vi "_complementStringArrays.vi"(9 "B":string[](array[string]), 10 "A":string[](array[string])) -> (2 "Result":string[](array[string]))   [LabVIEW 2013, in "tWorkerController.lvlib" / "tWorkerController.lvclass"]
doc: "Returns elements from A that don't exist in B."
uses:
  tWorkerController.lvclass
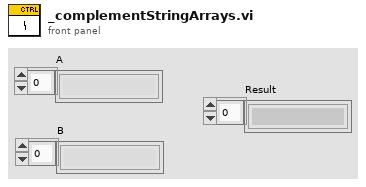
[diagram p1: front panel]
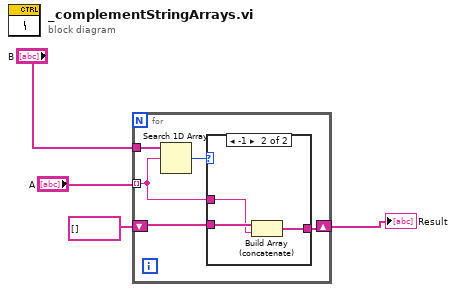
[diagram p0: block diagram]
diagram:
  n1 = for {
    tunnel: "A" -> [w7] mode=indexing
    shift-right: [w5] -> w1
    shift-left: string[] [] -> [w6]
    tunnel: "B" -> [w9]
    n2 = Search 1D Array(1D array=w9, element=w7) -> (index of element=w8:i32)  [unwired: 1 in]
    n3 = case shown="-1" w8 {
      tunnel: w7 -> [_ w12]
      tunnel: w6 -> [w10 w13]
      tunnel: [w10 w11] -> w5
      frame 0, Default {
      }
      frame -1 {
        n4 = Build Array (concatenate)(w13, w12) -> (w11:string[])
      }
    }
  }
  "Result" <- w1
